vi "RgbaToU32.vi"(11 "Rgba":T1) -> (3 "U32":u32)   [LabVIEW 2024, in "OpenLvVision_Image.lvlib" / "DataAccess.lvlib"]
doc: "Convert an color cluster into an number"
uses:
  DataAccess.lvlib
  TypeDef/RgbaU32.ctl
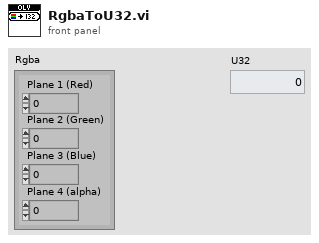
[diagram p1: front panel]
types:
  T1 = typedef "OpenLvVision_Image.lvlib/DataAccess.lvlib/RgbaU32.ctl" = cluster{"Plane 1 (Red)":u8, "Plane 2 (Green)":u8, "Plane 3 (Blue)":u8, "Plane 4 (alpha)":u8}
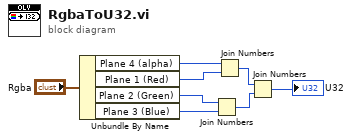
[diagram p0: block diagram]
diagram:
  n1 = Unbundle By Name("Rgba") -> ("Plane 4 (alpha)"=w4:u8, "Plane 1 (Red)"=w3:u8, "Plane 2 (Green)"=w2:u8, "Plane 3 (Blue)"=w1:u8)
  n2 = Join Numbers(hi=w2, lo=w1) -> ((hi.lo)=w6:u16)
  n3 = Join Numbers(hi=w4, lo=w3) -> ((hi.lo)=w7:u16)
  n4 = Join Numbers(hi=w7, lo=w6) -> ((hi.lo)=→"U32":u32)
